vi "frame_detector.vi"() -> ()   [LabVIEW 2010]
panel:
  out "error in (no error) 2":errorcluster
  out "VISA resource name 2":refnum<visa-resource-name>
  out "Array":i32[](array[numeric])
  in  "byte count":i32
  in  "error in (no error)":errorcluster
  in  "VISA resource name":refnum<visa-resource-name>
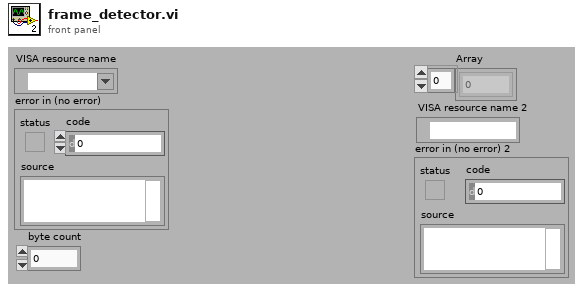
[diagram p1: front panel]
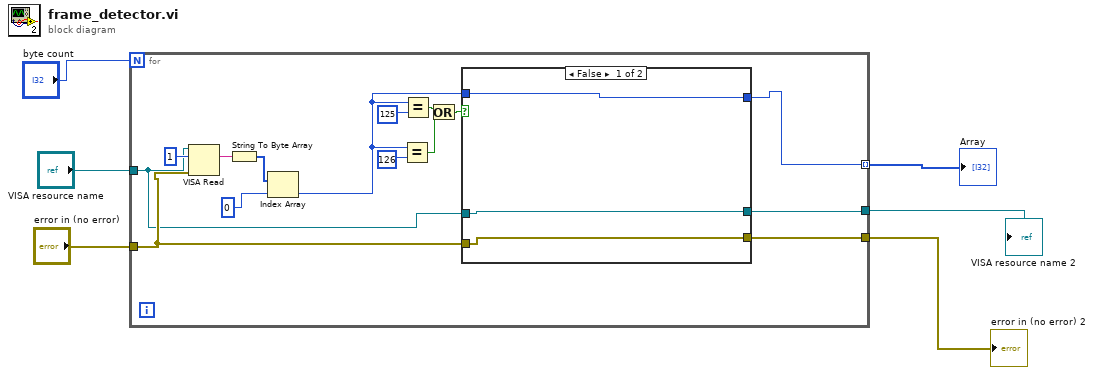
[diagram p0: block diagram]
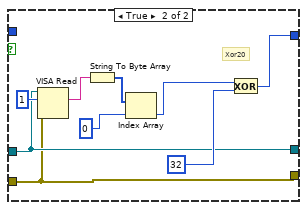
[diagram p2: hidden frame]
diagram:
  n1 = for {
    N: "byte count" -> [_]
    tunnel: "error in (no error)" -> [w11]
    tunnel: "VISA resource name" -> [w10]
    tunnel: [w9] -> w3 mode=indexing
    tunnel: [w8] -> w2
    tunnel: [w7] -> w1
    n2 = VISA Read(VISA resource name=w10, byte count=u32 1, error in (no error)=w11) -> (read buffer=w15:string)  [unwired: 3 out]
    n3 = String To Byte Array(string=w15) -> (unsigned byte array=w13:u8[])
    n4 = Index Array(array=w13, index=0) -> (element=w12:u8)
    n5 = Equal?(x=w12, y=u16 126) -> (x = y?=w19:bool)
    n6 = Equal?(x=w12, y=u16 125) -> (x = y?=w18:bool)
    n7 = Or(x=w18, y=w19) -> (x .or. y?=w17:bool)
    n8 = case shown="False" w17 {
      tunnel: w12 -> [w24 _]
      tunnel: [w24 w32] -> w9
      tunnel: w10 -> [w23 w26]
      tunnel: w11 -> [w22 w25]
      tunnel: [w23 w26] -> w8
      tunnel: [w22 w25] -> w7
      frame False {
      }
      frame True {
        # "Xor20"
        n9 = VISA Read(VISA resource name=w26, byte count=u32 1, error in (no error)=w25) -> (read buffer=w31:string)  [unwired: 3 out]
        n10 = String To Byte Array(string=w31) -> (unsigned byte array=w29:u8[])
        n11 = Index Array(array=w29, index=0) -> (element=w28:u8)
        n12 = Exclusive Or(1:32 ("y"), 2:w28) -> (0:w32:i32)
      }
    }
  }
  "Array" <- w3
  "VISA resource name 2" <- w2
  "error in (no error) 2" <- w1
